vi "test_Add Grouped Scalar Output Channels.vi"(8 "error in (no error)":errorcluster, 11 "TestCase in":refnum<class "FPGA Addon Adding Channel Items Unit Tests.lvclass">) -> (0 "error out":errorcluster, 3 "TestCase out":refnum<class "FPGA Addon Adding Channel Items Unit Tests.lvclass">)   [LabVIEW 2020, in "FPGA Addon Adding Channel Items Unit Tests.lvclass"]
uses:
  FPGA Addon Adding Channel Items Unit Tests.lvclass
  <vilib>/NI VeriStand/Custom Device API/Custom Device Channel.ctl
  <vilib>/NI VeriStand/Custom Device API/Custom Device Channel Type.ctl
  Addon/Addon System Explorer/Types/Channel Type.ctl
  Addon/Addon System Explorer/Types/SE UI Cluster.ctl
  <vilib>/NI VeriStand/Custom Device API/Custom Device Item Ref.ctl
  FPGA Addon Adding Channel Items Unit Tests.lvclass/FPGA Addon Adding Channel Items Unit Tests.ctl
  Addon/Addon Shared/SubVIs/Constants.vi
  <vilib>/NI VeriStand/Custom Device Tools/Custom Device Utility Library/NI VeriStand - Search for Item by GUID.vi
  <vilib>/NI/NI VeriStand Advanced SysDef API/_SubVIs/SysDef.Search.GUIDs.vi
  <vilib>/addons/_JKI Toolkits/VI Tester/TestCase.llb/TestCase.lvclass
  Addon/Addon System Explorer/FPGA Addon System Explorer.lvlib
  <vilib>/NI VeriStand/Custom Device Tools/Custom Device Utility Library/Custom Device Utility Library.lvlib
  Addon/Addon Shared/FPGA Addon Shared.lvlib
  <vilib>/NI/NI VeriStand Advanced SysDef API/SysDef API/Advanced System Definition.lvlib
  <vilib>/NI VeriStand/Custom Device API/Custom Device API.lvlib
  C:/Program Files (x86)/National Instruments/LabVIEW 2020/vi.lib/addons/_JKI Toolkits/VI Tester/TestCase.llb/TestCase.lvclass
panel:
  out "GUIDs":string[](array[string])
  out "Channels":T1[](array[typedef])
  in  "remove":bool
  in  "add":bool
  out "Names":string[](array[string])
  in  "Available Registers":i32[](listbox)
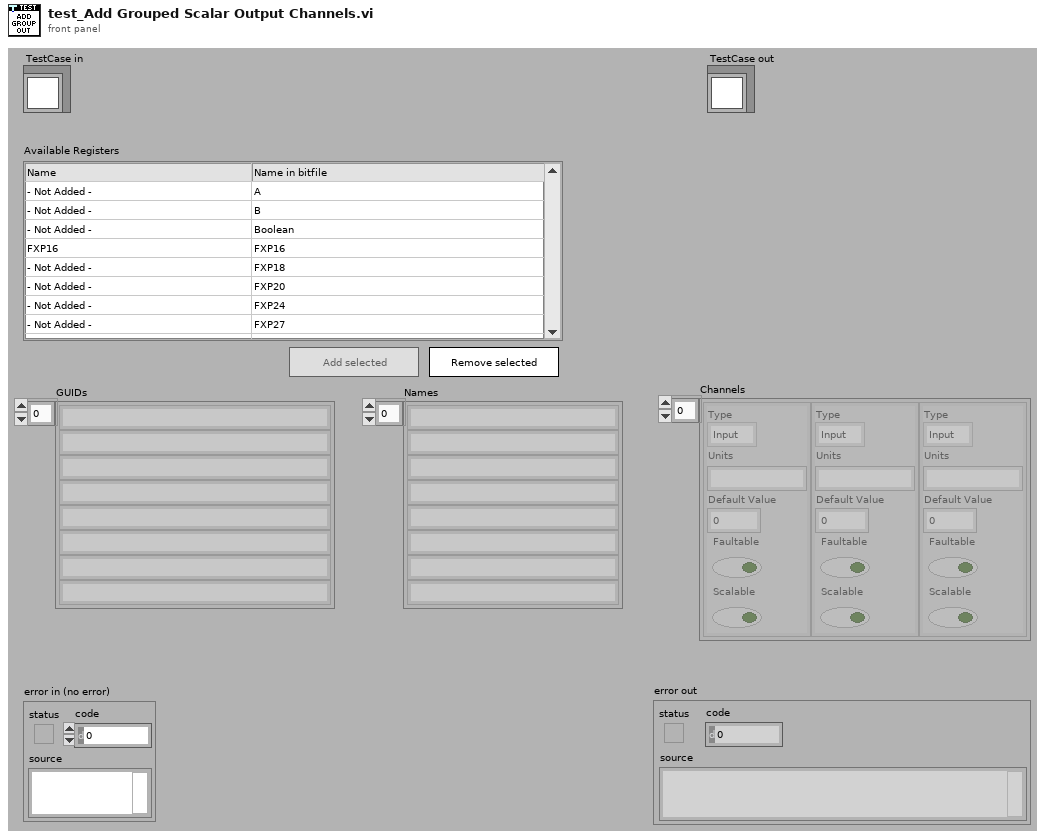
[diagram p1: front panel]
types:
  T1 = typedef "Custom Device API.lvlib/Custom Device Channel.ctl" = cluster{"Type":T2, "Units":string, "Default Value":dbl, "Faultable":bool, "Scalable":bool}
  T2 = typedef "Custom Device API.lvlib/Custom Device Channel Type.ctl" = enum16{"Input", "Output"}
  T3 = typedef "FPGA Addon System Explorer.lvlib/SE UI Cluster.ctl" = cluster{"Node Ptr":T4, "Add":refnum<vi>, "Remove":refnum<vi>, "Registers ListBox":refnum<vi>}
  T4 = typedef "Custom Device API.lvlib/Custom Device Item Ref.ctl" = u64
  T5 = typedef "FPGA Addon System Explorer.lvlib/Channel Type.ctl" = enum16{"Write Channel", "Read Channel", "Write Waveform", "Read Waveform"}
  T6 = typedef "Advanced System Definition.lvlib/TreeItem.Info.ctl" = cluster{"Name":string, "Description":string, "GUID":string, "Is Channel":bool, "Channel":T1, "Is Waveform":bool, "Waveform":T7}
  T7 = typedef "Custom Device API.lvlib/Custom Device Waveform.ctl" = cluster{"Data Type":T8, "Units":string}
  T8 = typedef "Custom Device API.lvlib/Custom Device Waveform DataType.ctl" = enum16{"Double", "Complex Double"}
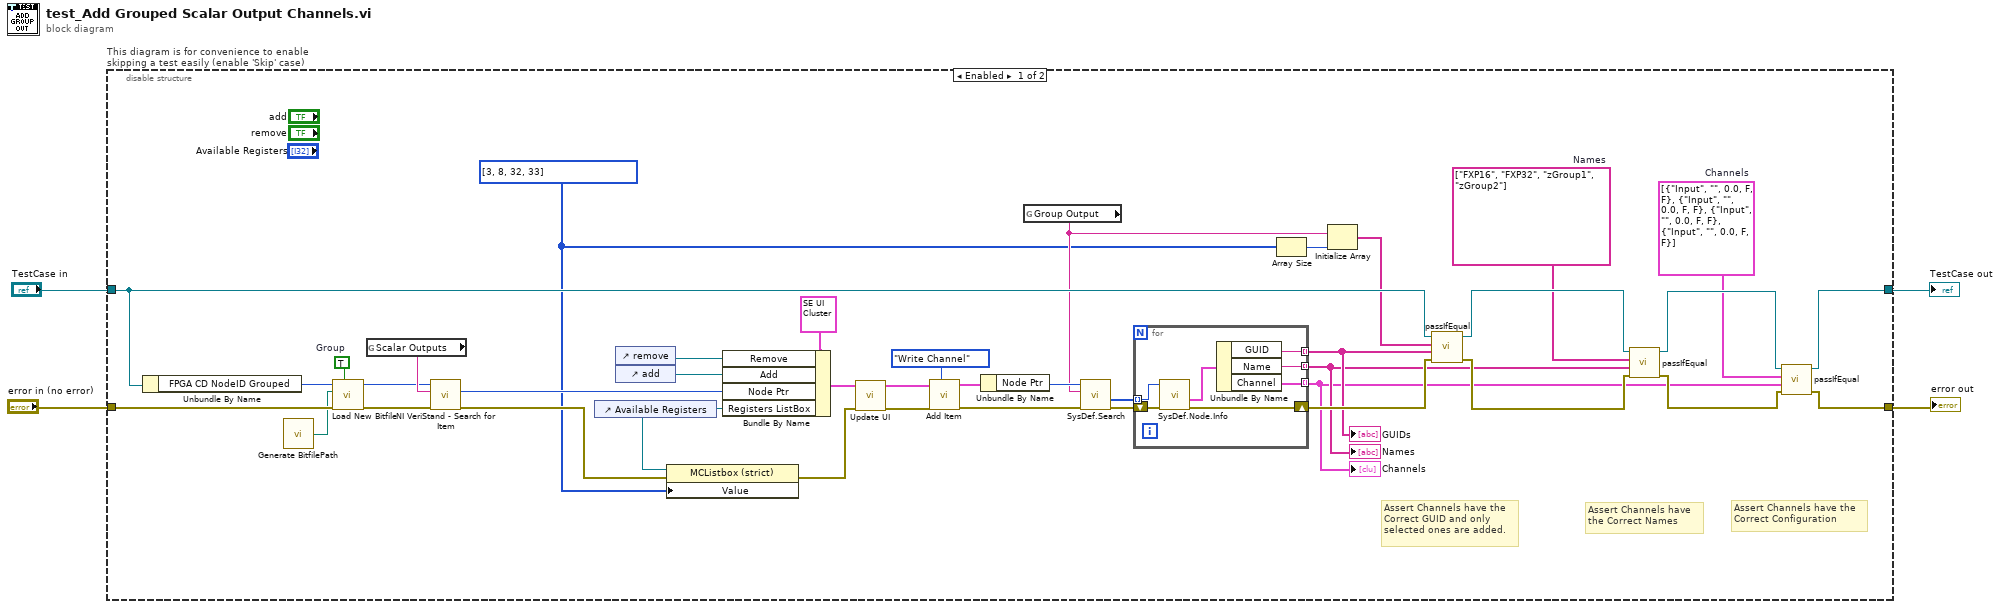
[diagram p0: block diagram]
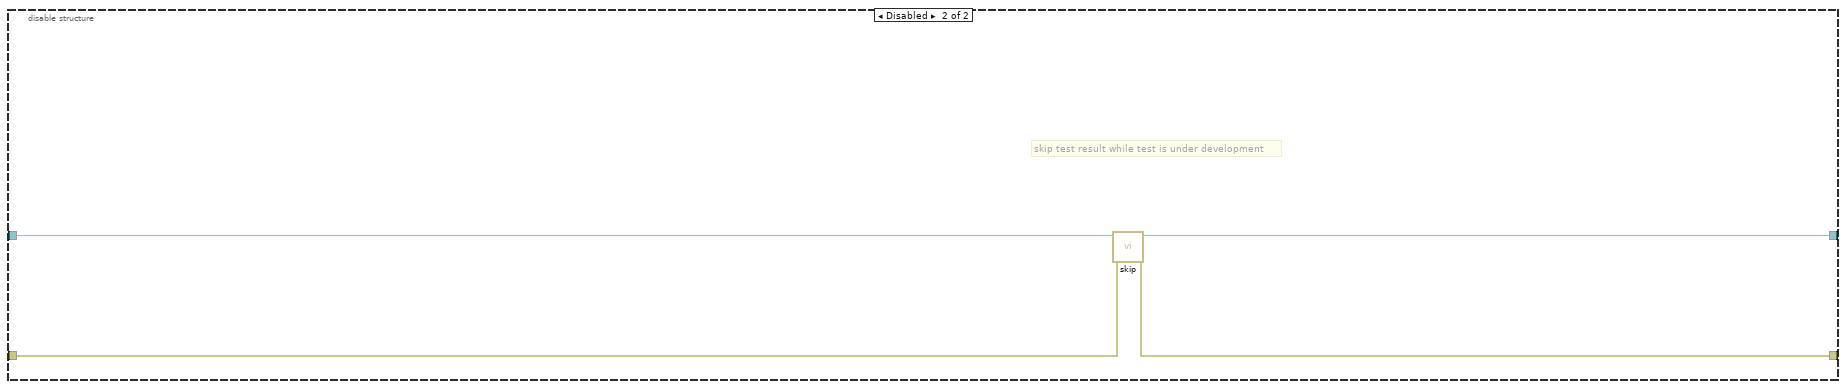
[diagram p2: hidden frame]
diagram:
  n1 = disable-structure "This diagram is for convenience to enable skipping a test easily (enable 'Skip' case)" shown="Enabled" {
    disable-tunnel: "TestCase in" -> [w36 w55]
    disable-tunnel: [w32 w53] -> w1
    disable-tunnel: [w29 w54] -> w3
    disable-tunnel: "error in (no error)" -> [w25 w52]
    frame Enabled {
      w16 = TRUE  # Group
      w27 = T1[] [{"Type"=enum."Input", "Units"="", "Default Value"=0.0, "Faultable"=FALSE, "Scalable"=FALSE}, {"Type"=enum."Input", "Units"="", "Default Value"=0.0, "Faultable"=FALSE, "Scalable"=FALSE}, {"Type"=enum."Input", "Units"="", "Default Value"=0.0, "Faultable"=FALSE, "Scalable"=FALSE}, {"Type"=enum."Input", "Units"="", "Default Value"=0.0, "Faultable"=FALSE, "Scalable"=FALSE}]  # Channels
      w33 = string[] ["FXP16", "FXP32", "zGroup1", "zGroup2"]  # Names
      w6 = i32[] [3, 8, 32, 33] ("selected")
      # "Assert Channels have the Correct Configuration"
      # "Assert Channels have the Correct Names"
      # "Assert Channels have the Correct GUID and only selected ones are added."
      n2 = Unbundle By Name(w36) -> ("FPGA CD NodeID Grouped"=w24:u64)
      n3 = call "Generate BitfilePath.vi"() -> ("Bitfile path"=w23:path)
      n4 = call "Load New Bitfile.vi"("Group"=w16, "error in (no error)"=w25, "NewVal"=w23, "Item Ref in"=w24) -> ("error out"=w26:errorcluster, "Section Ref out"=w22:T4)  [unwired: 6 in]
      n5 = global read "Constants.vi" "Scalar Outputs"() -> (w43:string)
      n6 = call-poly <vilib>:"NI VeriStand - Search for Item.vi"("error in"=w26, "Item GUID"=w43, "Section Ref in"=w22) -> ("error out"=w7:errorcluster, "Item Ref"=w12:T4)  [unwired: 5 in, 2 out]
      n7 = control-ref of="Available Registers"() -> (w8:refnum<vi>)
      n8 = control-ref of="remove"() -> (w10:refnum<vi>)
      n9 = control-ref of="add"() -> (w9:refnum<vi>)
      n10 = property class="MCListbox (strict)"(reference=w8, error in=w7, "Value"=w6) -> (error out=w5:errorcluster)  [unwired: 1 out]
      n11 = Bundle By Name(cluster=T3 {"Node Ptr"=18446744073709551615, "Add"=refnum, "Remove"=refnum, "Registers ListBox"=refnum} ("SE UI cluster in"), "Remove"=w10, "Add"=w9, "Node Ptr"=w12, "Registers ListBox"=w8) -> (w11:T3)
      n12 = call "Update UI.vi"("error in (no error)"=w5, "SE UI cluster in"=w11) -> ("error out"=w15:errorcluster, "SE UI cluster out"=w14:T3)  [unwired: 8 in]
      n13 = call "Add Item.vi"("Action"=Channel_Type."Write Channel", "error in (no error)"=w15, "SE UI cluster in"=w14) -> ("error out"=w21:errorcluster, "SE UI cluster out"=w20:T3)  [unwired: 7 in]
      n14 = Unbundle By Name(w20) -> ("Node Ptr"=w41:T4)
      n15 = global read "Constants.vi" "Group Output"() -> (w18:string)
      n16 = call-poly <vilib>:"SysDef.Search.vi"("error in (no error)"=w21, "GUID"=w18, "nodeID"=w41) -> ("error out"=w42:errorcluster, "Values Out"=w40:u64[])  [unwired: 5 in, 2 out]
      n17 = for {
        tunnel: w40 -> [w47] mode=indexing
        tunnel: [w45] -> w34 mode=indexing
        tunnel: [w48] -> w28 mode=indexing
        tunnel: [w46] -> w37 mode=indexing
        shift-right: [w50] -> w38
        shift-left: w42 -> [w51]
        n18 = call <vilib>:"SysDef.Node.Info.vi"("error in (no error)"=w51, "nodeID"=w47) -> ("error out"=w50:errorcluster, "Item Info"=w49:T6)  [unwired: 6 in, 2 out]
        n19 = Unbundle By Name(w49) -> ("GUID"=w46:string, "Name"=w45:string, "Channel"=w48:T1)
      }
      "Names" <- w34
      "Channels" <- w28
      "GUIDs" <- w37
      n20 = Array Size(array=w6) -> (size(s)=w17:i32)
      n21 = Initialize Array(w18, w17) -> (w19:string[])
      n22 = call-dynamic "passIfEqual.vi"("error in (no error)"=w38, "y"=w37, "x"=w19, "TestCase in"=w36) -> ("error out"=w39:errorcluster, "TestCase out"=w35:refnum<class "FPGA Addon Adding Channel Items Unit Tests.lvclass">)  [unwired: 6 in]
      n23 = call-dynamic "passIfEqual.vi"("error in (no error)"=w39, "y"=w34, "x"=w33, "TestCase in"=w35) -> ("error out"=w30:errorcluster, "TestCase out"=w31:refnum<class "FPGA Addon Adding Channel Items Unit Tests.lvclass">)  [unwired: 6 in]
      n24 = call-dynamic "passIfEqual.vi"("error in (no error)"=w30, "y"=w28, "x"=w27, "TestCase in"=w31) -> ("error out"=w29:errorcluster, "TestCase out"=w32:refnum<class "FPGA Addon Adding Channel Items Unit Tests.lvclass">)  [unwired: 6 in]
    }
    frame Disabled {
      # "skip test result while test is under development"
      n25 = call <vilib>:"skip.vi"("error in (no error)"=w52, "TestCase in"=w55) -> ("error out"=w54:errorcluster, "TestCase out"=w53:refnum<class "FPGA Addon Adding Channel Items Unit Tests.lvclass">)  [unwired: 8 in]
    }
  }
  "error out" <- w3
  "TestCase out" <- w1
